vi "DecodeNumericFrame.vi"(8 "ErrorIn":errorcluster, 11 "Frame":string) -> (0 "ErrorOut":errorcluster, 3 "ReceivedValue":u32)   [LabVIEW 2016]
doc: "Decode data frame in order to get number of measument packets available to read.\n\nIf there is an arror during processing or at the input, VI ends execution and throws error."
uses:
  DecodeNumericFrame/DNFDataFrameSection.ctl
  DecodeNumericFrame/DNFContext.ctl
  DecodeNumericFrame/DNFDataFrameSectionsLen.ctl
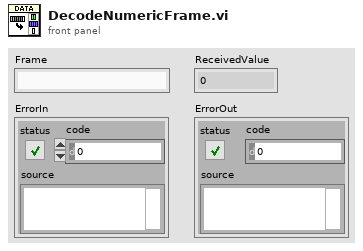
[diagram p1: front panel]
types:
  T1 = typedef "DNFDataFrameSectionsLen.ctl" = cluster{"Header":i32, "Data":i32}
  T2 = typedef "DNFContext.ctl" = cluster{"Frame":string, "FrameHeader":string, "DataFrameSectionsLen":cluster{"Header":i32, "Data":i32}, "ReceivedValue":u32}
  T3 = typedef "DNFDataFrameSection.ctl" = enum16{"SOF", "Header", "Data", "EOF"}
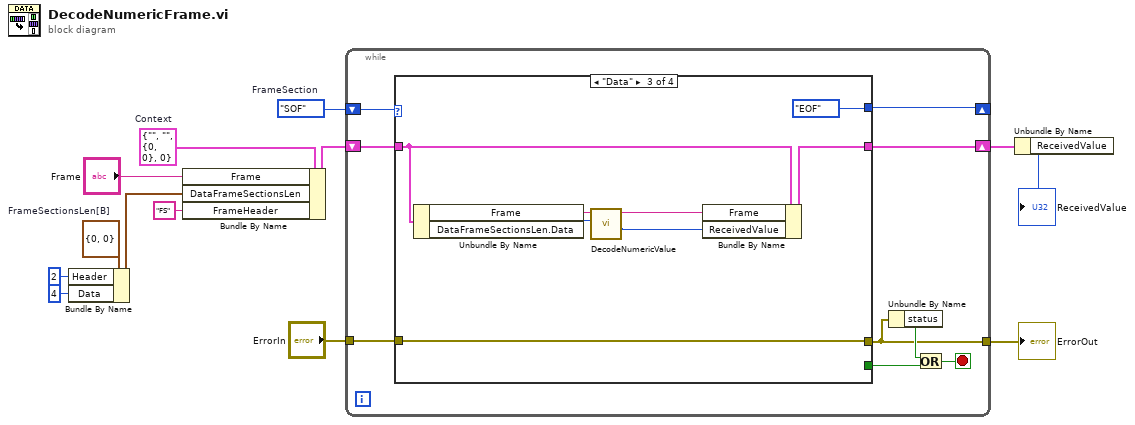
[diagram p0: block diagram]
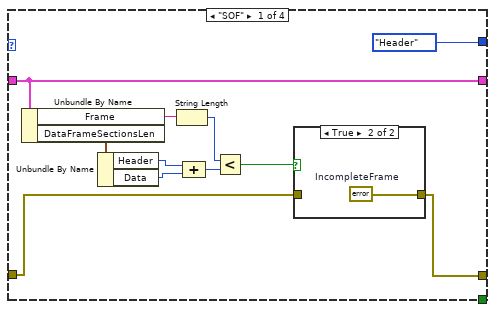
[diagram p2: hidden frame]
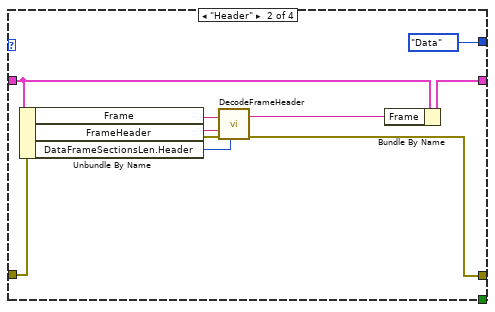
[diagram p4: hidden frame]
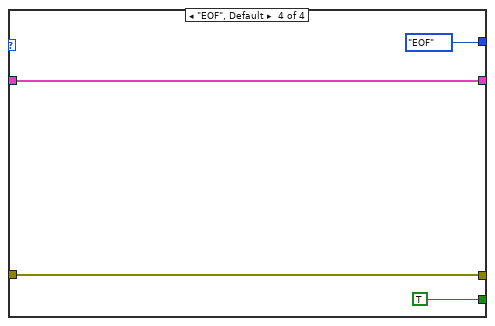
[diagram p5: hidden frame]
diagram:
  w1 = T1 {"Header"=0, "Data"=0}  # FrameSectionsLen[B]
  w2 = T2 {"Frame"="", "FrameHeader"="", "DataFrameSectionsLen"={"Header"=0, "Data"=0}, "ReceivedValue"=0}  # Context
  w3 = DNFDataFrameSection."SOF"  # FrameSection
  n1 = Bundle By Name(cluster=w1, "Header"=2, "Data"=4) -> (w9:T1)
  n2 = Bundle By Name(cluster=w2, "Frame"="Frame", "DataFrameSectionsLen"=w9, "FrameHeader"="FS") -> (w11:T2)
  n3 = while {
    shift-right: [w14] -> _
    shift-left: w3 -> [w15]
    shift-right: [w20] -> w5
    shift-left: w11 -> [w22]
    tunnel: "ErrorIn" -> [w21]
    tunnel: [w16] -> w6
    stop <- w19 stop-if-true
    n4 = case shown="\"Data\"" w15 {
      tunnel: w22 -> [w25 w41 w49 w54]
      tunnel: w21 -> [w26 w42 w47 w55]
      tunnel: [w25 w39 w48 w54] -> w20
      tunnel: [DNFDataFrameSection."Header" ("FrameSection") DNFDataFrameSection."Data" ("FrameSection") DNFDataFrameSection."EOF" ("FrameSection") DNFDataFrameSection."EOF" ("FrameSection")] -> w14
      tunnel: [w24 w38 w47 w55] -> w16
      tunnel: [_ _ _ TRUE] -> w17
      frame "SOF" {
        n5 = Unbundle By Name(w25) -> ("Frame"=w33:string, "DataFrameSectionsLen"=w32:cluster{"Header":i32, "Data":i32})
        n6 = Unbundle By Name(w32) -> ("Header"=w31:i32, "Data"=w30:i32)
        n7 = String Length(string=w33) -> (length=w29:i32)
        n8 = Compound Arithmetic op=ADD(w31, w30) -> (w28:i32)
        n9 = Less?(x=w29, y=w28) -> (x < y?=w27:bool)
        n10 = case shown="True" w27 {
          tunnel: w26 -> [w34 _]
          tunnel: [w34 w35] -> w24
          frame False {
          }
          frame True {
            w35 = errorcluster {"status"=TRUE, "code"=1, "source"="Incomplete frame"}  # IncompleteFrame
          }
        }
      }
      frame "Header" {
        n11 = Unbundle By Name(w41) -> ("Frame"=w43:string, "FrameHeader"=w44:string, "DataFrameSectionsLen.Header"=w37:i32)
        n12 = call "DecodeFrameHeader.vi"("HeaderLen"=w37, "ErrorIn"=w42, "Header"=w44, "Frame"=w43) -> ("ErrorOut"=w38:errorcluster, "Remainder"=w40:string)  [unwired: 5 in, 1 out]
        n13 = Bundle By Name(cluster=w41, "Frame"=w40) -> (w39:T2)
      }
      frame "Data" {
        n14 = Unbundle By Name(w49) -> ("Frame"=w50:string, "DataFrameSectionsLen.Data"=w51:i32)
        n15 = call "DecodeNumericValue.vi"("DataLen"=w51, "Frame"=w50) -> ("NumericValue"=w45:u32, "Remainder"=w52:string)  [unwired: 8 in]
        n16 = Bundle By Name(cluster=w49, "Frame"=w52, "ReceivedValue"=w45) -> (w48:T2)
      }
      frame "EOF", Default {
      }
    }
    n17 = Unbundle By Name(w16) -> ("status"=w18:bool)
    n18 = Or(x=w18, y=w17) -> (x .or. y?=w19:bool)
  }
  "ErrorOut" <- w6
  n19 = Unbundle By Name(w5) -> ("ReceivedValue"=→"ReceivedValue":u32)
